vi "VdAnalogInput_Simulated_Create.vi"(6 "VoltageRangeHigh":dbl, 8 "Error In":errorcluster, 9 "VoltageRangeLow":dbl, 10 "Address":string, 11 "reference in":refnum<class "VdAnalogInput_Simulated.lvclass">) -> (0 "Error Out":errorcluster, 3 "reference out":refnum<class "VdAnalogInput_Simulated.lvclass">)   [LabVIEW 2020, in "VdAnalogInput_Simulated.lvclass"]
uses:
  VdAnalogInput_Simulated.lvclass
  VdAnalogInput_Simulated.lvclass/VdAnalogInput_Simulated.ctl
  VdAnalogInput_class/VdAnalogInput.lvclass
  C:/Projects/DesignPatterns/Factory1/VdAnalogInput_class/VdAnalogInput.lvclass
  C:/Projects/DesignPatterns/Factory1/VdInstrument_class/VdInstrument.lvclass
  C:/Projects/DesignPatterns/Factory1/VdAnalogInput_Simulated_class/VdAnalogInput_Simulated.lvclass
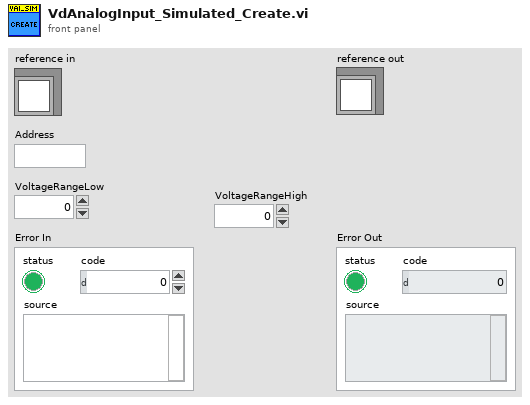
[diagram p1: front panel]
types:
  T1 = typedef "VdDigitalControl_Simulated.lvclass/ObjectAttributes.ctl" = cluster{"None":bool}
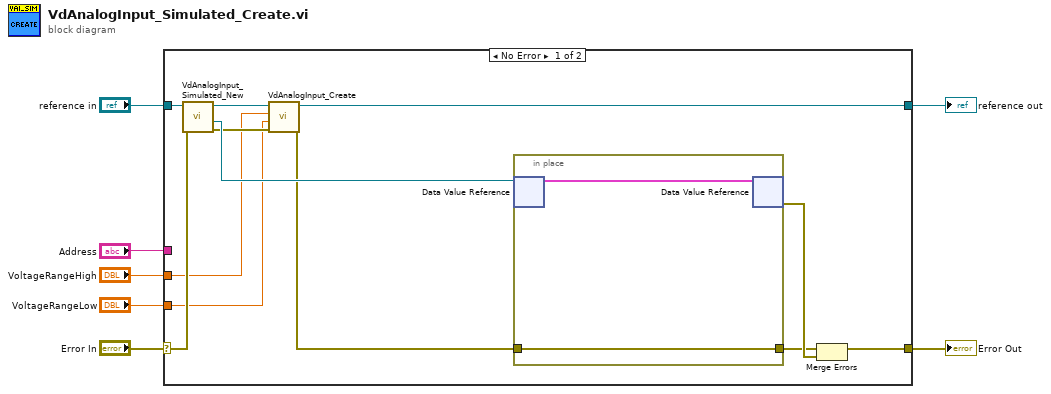
[diagram p0: block diagram]
diagram:
  n1 = case shown="No Error" "Error In" {
    selector: "Error In" -> [w15 w23]
    tunnel: [w13 w23] -> w6
    tunnel: "reference in" -> [w17 w22]
    tunnel: [w12 w22] -> w4
    tunnel: "Address" -> [_ _]
    tunnel: "VoltageRangeLow" -> [w9 _]
    tunnel: "VoltageRangeHigh" -> [w8 _]
    frame No Error {
      n2 = call "VdAnalogInput_Simulated_New.vi"("error in (no error)"=w15, "reference in"=w17) -> ("error out"=w16:errorcluster, "DVRRefOut"=w19:refnum<data-value>, "reference out"=w18:refnum<class "VdAnalogInput_Simulated.lvclass">)  [unwired: 6 in, 1 out]
      n3 = call "VdAnalogInput_Create.vi"("Error In"=w16, "VoltageRangeLow"=w9, "VoltageRangeHigh"=w8, "reference in"=w18) -> ("Error Out"=w10:errorcluster, "reference out"=w12:refnum<class "VdAnalogInput_Simulated.lvclass">)  [unwired: 6 in]
      n4 = in-place {
        in-place-border: w10 -> [w21]
        in-place-border: [w21] -> w11
        n5 = in-place-dvr #1(w19) -> (w20:T1)  [unwired: 1 out]
        n6 = in-place-dvr #1(w20) -> (w14:errorcluster)  [unwired: 1 out]
      }
      n7 = Merge Errors(w11, w14) -> (w13:errorcluster)
    }
    frame Error {
    }
  }
  "Error Out" <- w6
  "reference out" <- w4
